vi "Post-Install Action.vi"() -> ()   [LabVIEW 2022 SP3]
panel:
  in  "go":bool
  # "gScript requires that the Aerotech libraries are copied into it's install directory. Click the button\nbelow to copy these files automatically."
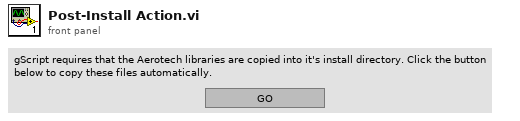
[diagram p1: front panel]
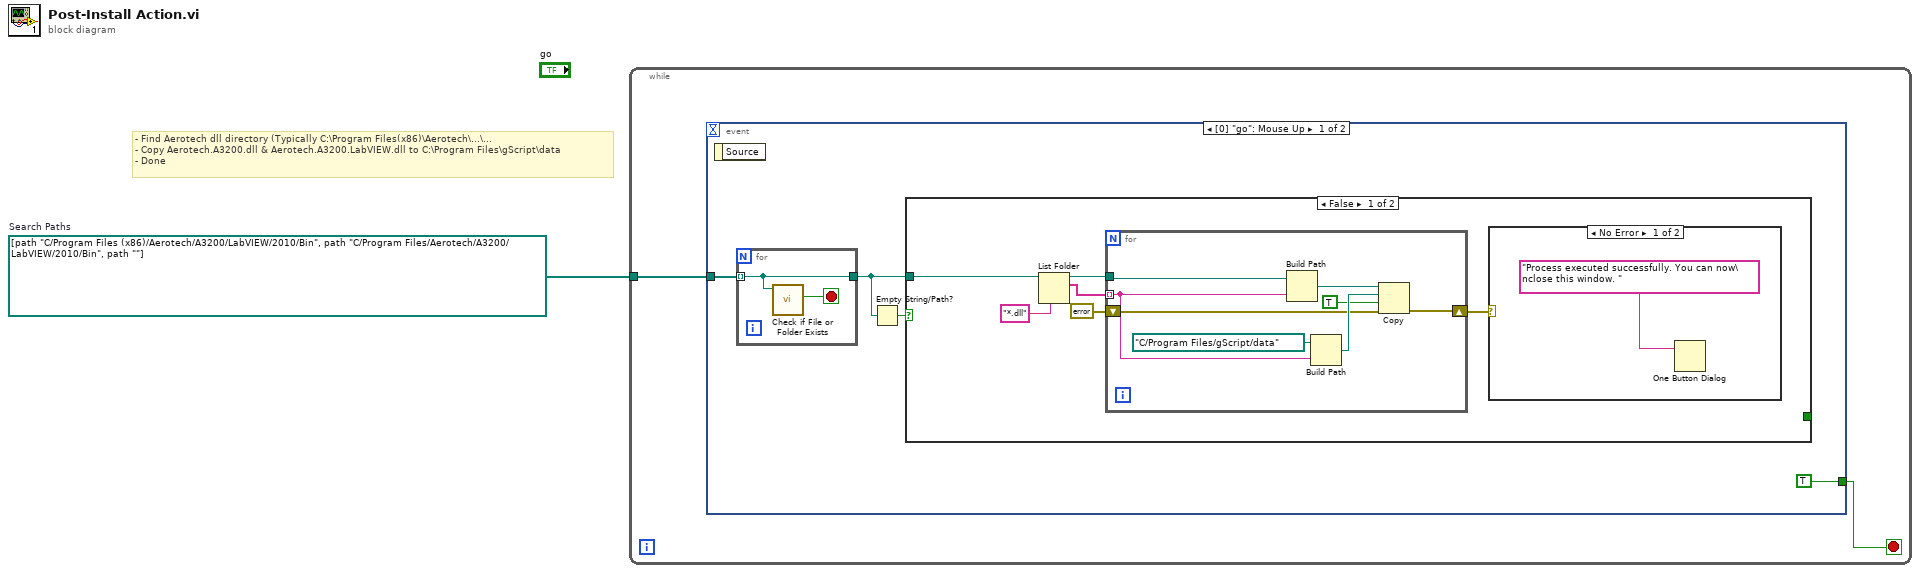
[diagram p0: block diagram]
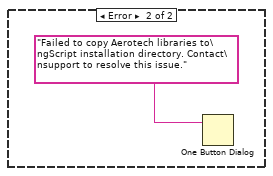
[diagram p2: hidden frame]
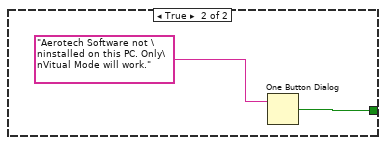
[diagram p3: hidden frame]
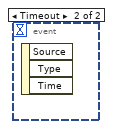
[diagram p4: hidden frame]
diagram:
  w1 = path[] [path "C:/Program Files (x86)/Aerotech/A3200/LabVIEW/2010/Bin", path "C:/Program Files/Aerotech/A3200/LabVIEW/2010/Bin", path ""]  # Search Paths
  # "- Find Aerotech dll directory (Typically C:\\Program Files(x86)\\Aerotech\\...\\...\n- Copy Aerotech.A3200.dll & Aerotech.A3200.LabVIEW.dll to C:\\Program Files\\gScript\\data\n- Done"
  n1 = while {
    tunnel: w1 -> [w3]
    stop <- w2 stop-if-true
    n2 = event shown="[0] \"go\": Mouse Up" {
      selector: _ -> [_ _]
      dyn-events: _ -> [_ _]
      timeout: _ -> [_ _]
      tunnel: w3 -> [w7 _]
      tunnel: [TRUE _] -> w2
      event "go": Mouse Up {
        n3 = event-data() -> ()  [unwired: 1 in, 1 out]
        n4 = for {
          tunnel: w7 -> [w26] mode=indexing
          tunnel: [w26] -> w5
          stop <- w27 stop-if-true
          n5 = call <vilib>:"Check if File or Folder Exists.vi"("path"=w26) -> ("file or folder exists?"=w27:bool)  [unwired: 8 in, 2 out]
        }
        n6 = Empty String/Path?(string/path=w5) -> (empty?=w6:bool)
        n7 = case shown="False" w6 {
          tunnel: w5 -> [w11 _]
          tunnel: [_ w24] -> _
          frame False {
            n8 = List Folder(path=w11, pattern="*.dll") -> (path out=w10:path, filenames=w8:string[])  [unwired: 2 in, 2 out]
            n9 = for {
              tunnel: w10 -> [w23]
              shift-right: [w18] -> w12
              shift-left: errorcluster {"status"=FALSE, "code"=0, "source"=""} ("error out") -> [w17]
              tunnel: w8 -> [w16] mode=indexing
              n10 = Build Path(base path=w23, name or relative path=w16) -> (appended path=w22:path)
              n11 = Build Path(base path=path "C:/Program Files/gScript/data", name or relative path=w16) -> (appended path=w20:path)
              n12 = Copy(8:w17, 9:TRUE ("overwrite (F)"), 10:w20, 11:w22) -> (0:w18:errorcluster)  [unwired: 1 in, 2 out]
            }
            n13 = case shown="No Error" w12 {
              frame No Error {
                n14 = One Button Dialog(message="Process executed successfully. You can now\nclose this window. ") -> ()  [unwired: 1 in, 1 out]
              }
              frame Error {
                n15 = One Button Dialog(message="Failed to copy Aerotech libraries to\ngScript installation directory. Contact\nsupport to resolve this issue.") -> ()  [unwired: 1 in, 1 out]
              }
            }
          }
          frame True {
            n16 = One Button Dialog(message="Aerotech Software not \ninstalled on this PC. Only\nVitual Mode will work.") -> (true=w24:bool)  [unwired: 1 in]
          }
        }
      }
      event Timeout {
        n17 = event-data() -> ()  [unwired: 1 in, 3 out]
      }
    }
  }
